vi "oax_Tacho Channel Warning.vi"(8 "error in (no error)":errorcluster, 11 "Channels":bool[](array[boolean])=[FALSE, FALSE, TRUE, FALSE, FALSE, FALSE, FALSE, FALSE]) -> (0 "error out":errorcluster, 3 "tachometer channel 2":u16(ring)=2 items=["ch 0", "ch 1", "ch 2", "ch 3", "ch 4", "ch 5", "ch 6", "ch 7"])   [LabVIEW 2017]
panel:
  in  "Stop":bool
  in  "tachometer channel":u16(ring)
  # "Incorrect tachometer channel selection!"
  # "The tachometer channel is not selected in Channels selection"
  # "Select the correct tachometer channel:"
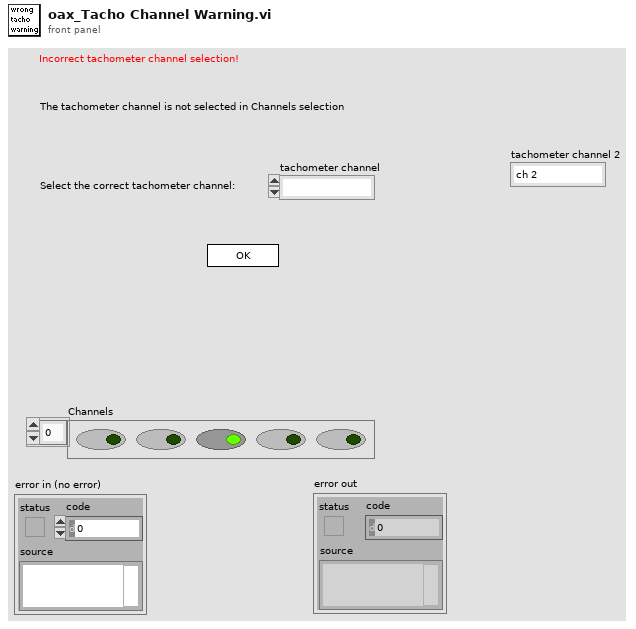
[diagram p1: front panel]
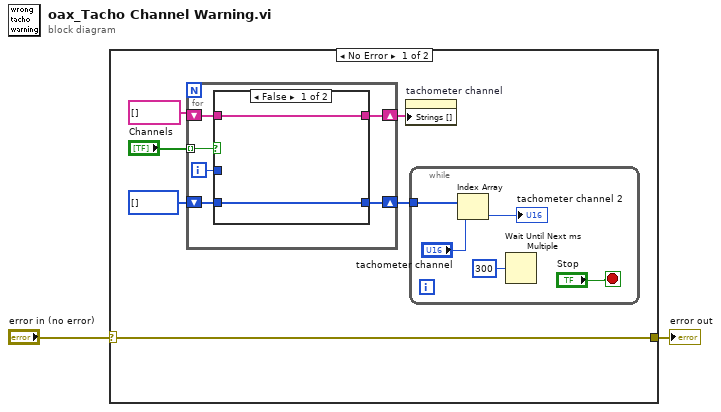
[diagram p0: block diagram]
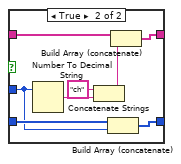
[diagram p2: hidden frame]
diagram:
  n1 = case shown="No Error" "error in (no error)" {
    selector: "error in (no error)" -> [w4 w30]
    tunnel: [w4 w30] -> w1
    frame No Error {
      n2 = for {
        tunnel: "Channels" -> [w19] mode=indexing
        shift-right: [w17] -> w6
        shift-left: string[] [] -> [w16]
        shift-right: [w14] -> w3
        shift-left: i32[] [] -> [w15]
        i -> [w18]
        n3 = case shown="False" w19 {
          tunnel: w18 -> [_ w23]
          tunnel: [w21 w27] -> w17
          tunnel: w16 -> [w21 w26]
          tunnel: w15 -> [w20 w24]
          tunnel: [w20 w22] -> w14
          frame False {
          }
          frame True {
            n4 = Number To Decimal String(number=w23) -> (decimal integer string=w28:string)  [unwired: 1 in]
            n5 = Concatenate Strings("ch" ("string"), w28) -> (w25:string)
            n6 = Build Array (concatenate)(w24, w23) -> (w22:i32[])
            n7 = Build Array (concatenate)(w26, w25) -> (w27:string[])
          }
        }
      }
      n8 = property on="tachometer channel" class="Ring (strict)"("Strings []"=w6) -> ()  [unwired: 2 in, 2 out]
      n9 = while {
        tunnel: w3 -> [w11]
        stop <- "Stop" stop-if-true
        n10 = Index Array(array=w11, index="tachometer channel") -> (element=→"tachometer channel 2":i32)
        n11 = Wait Until Next ms Multiple(millisecond multiple=u32 300) -> ()  [unwired: 1 out]
      }
    }
    frame Error {
    }
  }
  "error out" <- w1
